vi "CreateEpub.vi"(6 "线程":i32=4, 8 "error in (no error)":errorcluster caption="错误输入（无错误）", 11 "EPUB 输入":refnum<class "EPUB.lvclass">) -> (0 "error out":errorcluster caption="错误输出", 3 "EPUB 输出":refnum<class "EPUB.lvclass">)   [LabVIEW 2016, in "EPUB.lvclass"]
uses:
  EPUB.lvclass
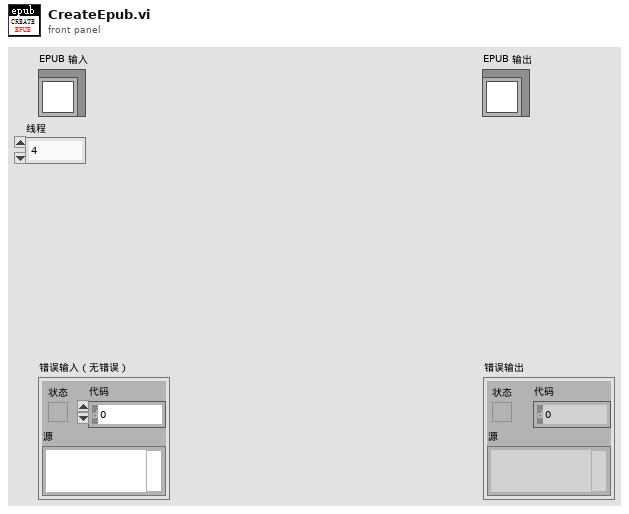
[diagram p1: front panel]
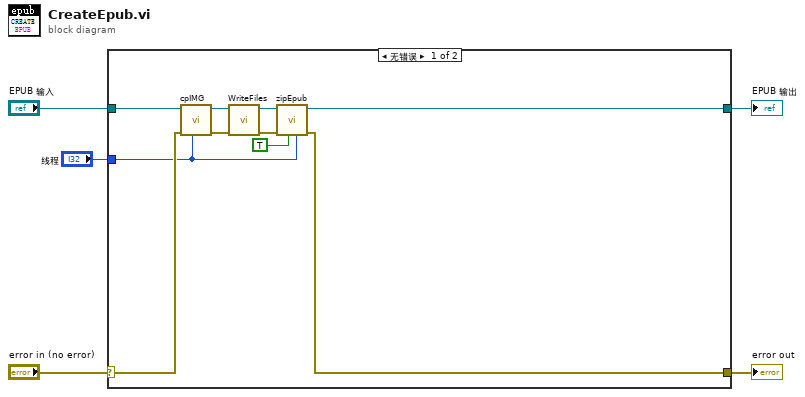
[diagram p0: block diagram]
diagram:
  n1 = case shown="无错误" "error in (no error)" {
    selector: "error in (no error)" -> [w8 w17]
    tunnel: [w7 w17] -> w4
    tunnel: [w11 w16] -> w2
    tunnel: "EPUB 输入" -> [w14 w16]
    tunnel: "线程" -> [w6 _]
    frame No Error {
      n2 = call "cpIMG.vi"("线程"=w6, "error in (no error)"=w8, "EPUB 输入"=w14) -> ("error out"=w12:errorcluster, "EPUB 输出"=w15:refnum<class "EPUB.lvclass">)  [unwired: 7 in]
      n3 = call "WriteFiles.vi"("error in (no error)"=w12, "EPUB 输入"=w15) -> ("error out"=w10:errorcluster, "EPUB 输出"=w13:refnum<class "EPUB.lvclass">)  [unwired: 8 in]
      n4 = call "zipEpub.vi"("线程"=w6, "删除临时文件"=TRUE, "error in (no error)"=w10, "EPUB 输入"=w13) -> ("error out"=w7:errorcluster, "EPUB 输出"=w11:refnum<class "EPUB.lvclass">)  [unwired: 6 in]
    }
    frame Error {
    }
  }
  "error out" <- w4
  "EPUB 输出" <- w2
